vi "Drag to Tree Check.vi"(6 "CtlRef":refnum<vi>, 7 "Coords":T1, 8 "Error In":errorcluster, 9 "Other names to check":string[](array[string])=["LV_LISTBOX_ITEMS"], 10 "Name source":string="LV_TEXT", 11 "Available Data Names":string[](array[string])) -> (0 "Error Out":errorcluster, 1 "Tag":string, 2 "Valid":bool, 3 "Name":string, 4 "Others valid":bool)   [LabVIEW 2016]
uses:
  <vilib>/Utility/miscctls.llb/LVPoint32TypeDef.ctl
panel:
  out "In Symbol?":bool
  out "In Bounds?":bool
  out "Column":i32
  out "Tree tag":string
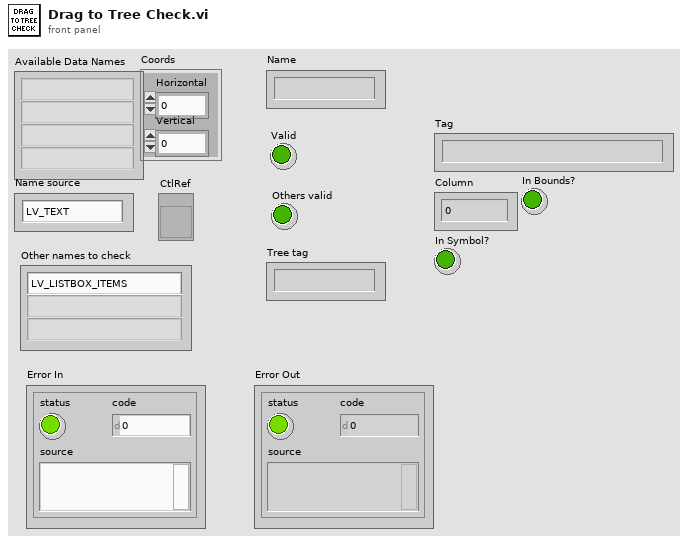
[diagram p1: front panel]
types:
  T1 = typedef "LVPoint32TypeDef.ctl" = cluster{"Horizontal":i32, "Vertical":i32}
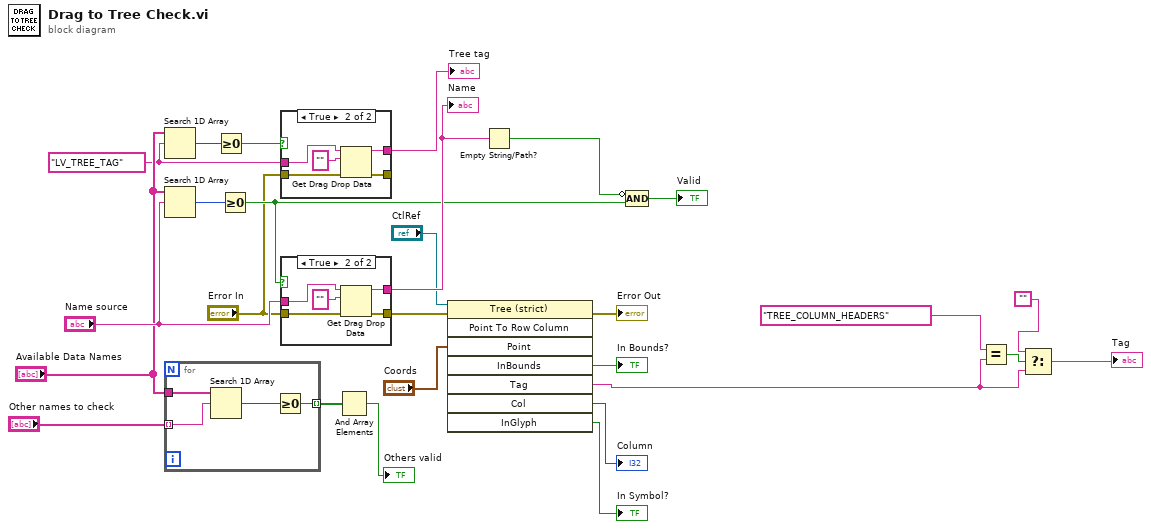
[diagram p0: block diagram]
diagram:
  w14 = "LV_TREE_TAG"
  n1 = Search 1D Array(1D array="Available Data Names", element=w14) -> (index of element=w17:i32)  [unwired: 1 in]
  n2 = Search 1D Array(1D array="Available Data Names", element="Name source") -> (index of element=w27:i32)  [unwired: 1 in]
  n3 = for {
    tunnel: "Available Data Names" -> [w31]
    tunnel: "Other names to check" -> [w30] mode=indexing
    tunnel: [w28] -> w24 mode=indexing
    n4 = Search 1D Array(1D array=w31, element=w30) -> (index of element=w29:i32)  [unwired: 1 in]
    n5 = Greater Or Equal To 0?(x=w29) -> (x >= 0?=w28:bool)
  }
  n6 = Greater Or Equal To 0?(x=w17) -> (x >= 0?=w18:bool)
  n7 = Greater Or Equal To 0?(x=w27) -> (x >= 0?=w20:bool)
  n8 = case shown="True" w18 {
    tunnel: "Error In" -> [w32 w36]
    tunnel: [_ w35] -> w13
    tunnel: [w32 w34] -> _
    tunnel: w14 -> [_ w33]
    frame False {
    }
    frame True {
      n9 = Get Drag Drop Data(6:w36, 8:"", 9:w33) -> (0:w34:errorcluster, 3:w35:string)
    }
  }
  "Tree tag" <- w13
  n10 = case shown="True" w20 {
    tunnel: "Name source" -> [_ w43]
    tunnel: "Error In" -> [w38 w41]
    tunnel: [_ w40] -> w21
    tunnel: [w38 w39] -> w10
    frame False {
    }
    frame True {
      n11 = Get Drag Drop Data(6:w41, 8:"", 9:w43) -> (0:w39:errorcluster, 3:w40:string)
    }
  }
  "Name" <- w21
  n12 = And Array Elements(Boolean array=w24) -> (logical AND=→"Others valid":bool)
  n13 = invoke class="Tree (strict)" method="Point To Row Column"(reference="CtlRef", error in=w10, "Point"="Coords") -> (error out=→"Error Out":errorcluster, "InBounds"=→"In Bounds?":bool, "Tag"=w2:string, "Col"=→"Column":i32, "InGlyph"=→"In Symbol?":bool)  [unwired: 5 in, 3 out]
  n14 = Empty String/Path?(string/path=w21) -> (empty?=w22:bool)
  n15 = Compound Arithmetic op=AND(invert w22, w20) -> (→"Valid":bool)
  n16 = Equal?(x="TREE_COLUMN_HEADERS", y=w2) -> (x = y?=w4:bool)
  n17 = Select(t="", s=w4, f=w2) -> (s? t:f=→"Tag":string)
